vi "Recursively Delete Registry Key.vi"(6 "Registry View":T1 items=["Default"=0, "KEY_WOW64_64KEY"=8, "KEY_WOW64_32KEY"=9], 8 "error in (no error)":errorcluster, 10 "Subkey":string, 11 "root key (HKEY_LOCAL_MACHINE)":T2(ring)=enum."HKEY_LOCAL_MACHINE") -> (0 "error out":errorcluster)   [LabVIEW 2011]
uses:
  <vilib>/registry/registry.llb/Registry View.ctl
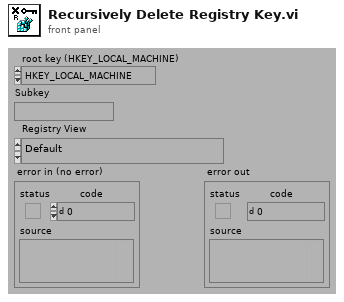
[diagram p1: front panel]
types:
  T1 = typedef "Registry View.ctl" = u16
  T2 = enum32{"HKEY_CLASSES_ROOT", "HKEY_CURRENT_USER", "HKEY_LOCAL_MACHINE", "HKEY_USERS", "HKEY_CURRENT_CONFIG"}
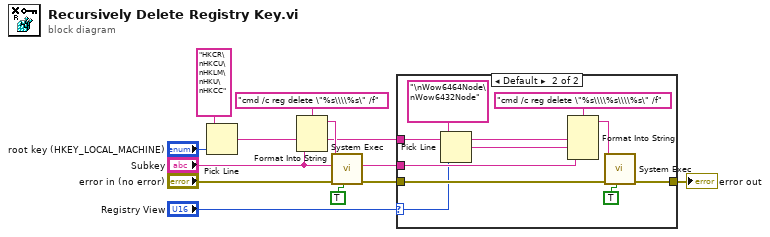
[diagram p0: block diagram]
diagram:
  n1 = Pick Line(multi-line string="HKCR\nHKCU\nHKLM\nHKU\nHKCC", line index="root key (HKEY_LOCAL_MACHINE)") -> (output string=w1:string)  [unwired: 1 in]
  n2 = Format Into String(format string="cmd /c reg delete \"%s\\\\%s\" /f" ("command line"), w1, "Subkey") -> (resulting string=w6:string)  [unwired: 2 in, 1 out]
  n3 = call <vilib>:"System Exec.vi"("run minimized? (F)"=TRUE, "error in (no error)"="error in (no error)", "command line"=w6) -> ("error out"=w4:errorcluster)  [unwired: 5 in, 3 out]
  n4 = case shown="Default" "Registry View" {
    selector: "Registry View" -> [_ w13]
    tunnel: w4 -> [w12 w18]
    tunnel: [w12 w17] -> w3
    tunnel: "Subkey" -> [_ w16]
    tunnel: w1 -> [_ w15]
    frame 0 {
    }
    frame Default {
      n5 = Pick Line(multi-line string="\nWow6464Node\nWow6432Node", line index=w13) -> (output string=w20:string)  [unwired: 1 in]
      n6 = Format Into String(format string="cmd /c reg delete \"%s\\\\%s\\\\%s\" /f" ("command line"), w15, w20, w16) -> (resulting string=w14:string)  [unwired: 2 in, 1 out]
      n7 = call <vilib>:"System Exec.vi"("run minimized? (F)"=TRUE, "error in (no error)"=w18, "command line"=w14) -> ("error out"=w17:errorcluster)  [unwired: 5 in, 3 out]
    }
  }
  "error out" <- w3
